vi "File Test Shell.vi"() -> (0 "error out":errorcluster, 3 "Test result":bool)   [LabVIEW 2018]
doc: "This VI is a shell to know how to call the class' test vi"
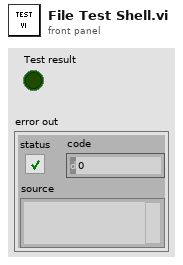
[diagram p1: front panel]
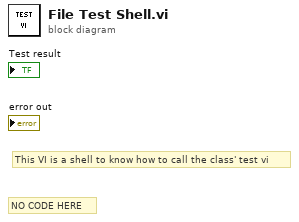
[diagram p0: block diagram]
diagram:
  # "NO CODE HERE"
  # "This VI is a shell to know how to call the class' test vi"
